vi "Soft_Robot_Model2.vi"() -> ()   [LabVIEW 2015]
uses:
  <vilib>/addons/Control Design/_Model Construction/Model Typedefs.llb/CD State Space Model (MIMO).ctl
  <vilib>/addons/Control Design/_Model Construction/Model Typedefs.llb/CD General Elements.ctl
  <vilib>/Platform/TimedLoop/XDataNode/timing_clust.ctl
  <vilib>/Platform/TimedLoop/XDataNode/nitl_modes.ctl
  <vilib>/Platform/TimedLoop/XDataNode/wakeup.ctl
  <vilib>/addons/Control Design/_Stochastic Systems/Stochastic Systems.llb/Stochastic Systems SubVIs/cd_Stochastic State-Space Model.ctl
  <vilib>/addons/Control Design/_Stochastic Systems/Stochastic Systems.llb/Stochastic Systems SubVIs/cd_Second-Order Statistics Noise Model.ctl
  <vilib>/addons/Control Design/_Model Construction/Model Creation.llb/Model Creation SubVI/cd_Create State Space Model.vi
  <vilib>/Simulation/Estimation/Implementation/NILVSim Discrete Kalman Filter.llb/SIM Disc KF Pred and Corr with Pred Gain with Checking Direct LV.vi
  <vilib>/addons/Control Design/_Implementation/CD State Feedback Controller (Multiple Outputs).vi
  <vilib>/FPGAPlugInAG/myRIO-1900/niLvFpga_Open_myRIO-1900.vi
  <vilib>/rvi/interface/common/dynamic/niFpgaDynamicAddResources.vi
  <vilib>/Utility/error.llb/Error Cluster From Error Code.vi
  <vilib>/rvi/errors/niLvFpgaAdjustHostInterfaceError.vi
  <vilib>/FPGAPlugInAG/Dynamic/niLvFpga_Close_Dynamic.vi
  <vilib>/Platform/TimedLoop/XDataNode/XDataNode.xnode
  <vilib>/Simulation/Implementation/XNodeFramework/SimXNode/SimX.xnode
  <vilib>/rvi/interface/nirviOpenFPGA/nirviOpenFPGA.xnode
  FPGA Bitfiles/ACC20115_FPGATarget_CurrentControlle_Dt5vFgOzYtY.lvbitx
  Current Controller.vi
  <vilib>/rvi/interface/nirviReadWriteControl/nirviReadWriteControl.xnode
  <vilib>/rvi/interface/nirviCloseFPGA/nirviCloseFPGA.xnode
  <vilib>/addons/Control Design/_Model Construction/NI_LinSys_Model Creation.lvlib
  <vilib>/Platform/TimedLoop/XDataNode/XDNodeRunTimeDep.lvlib
  NiFpgaLv.dll
  <vilib>/rvi/interface/Simulation/niFpgaSimulationCallBeginRW.vi
  <vilib>/addons/Control Design/_Implementation/NI_CD_Implementation.lvlib
  <vilib>/addons/Control Design/_Stochastic Systems/NI_CD_Stochastic Systems.lvlib
  <vilib>/addons/Control Design/_Model Construction/NI_LinSys_Model Typedefs.lvlib
panel:
  in  "SP":dbl(slide) scale=0.0..100.0
  in  "Tab Control":enum32{"Outputs", "Inputs"}(tab)
  out "Fusion Data":dbl(graph)
  out "KF Post":dbl[](graph)
  in  "Stop":bool
  out "DAC Inlet Valve 2":i32(graph)
  in  "Current (mA)":i32
  out "Status?":bool
  out "State-Space Model":T1={"properties"={"Model name"="", "Input names"=[], "Output names"=[], "Input Delays"=[], "Output Delays"=[], "Sampling Time"=0.0, "Notes"=""}, "A"=[], "B"=[[3.03e-07], [4.04e-07]], "C"=[], "D"=[], "StateNames"=[], "Transport Delay"=[]} {"Transport Delay" format="%.2f"; "D" format="%#.2g"; "C" format="%#.2g"; "B" format="%#.2g"; "A" format="%#.2g"; "properties"."Sampling Time" format="%#.6p"; "properties"."Output Delays" format="%.4f"; "properties"."Input Delays" format="%.4f"}
  out "KF Gain M(k)":dbl[][](array[numeric])
  in  "A":dbl[][](array[numeric])=[[1.01, -0.1716], [0.001556, 0.9782]] format="%#.5g"
  in  "B":dbl[][](array[numeric]) format="%#.5g"
  in  "C":dbl[][](array[numeric])=[[1.089, -0.03769]] format="%#.5g"
  out "error out":errorcluster
  out "KF Error":errorcluster
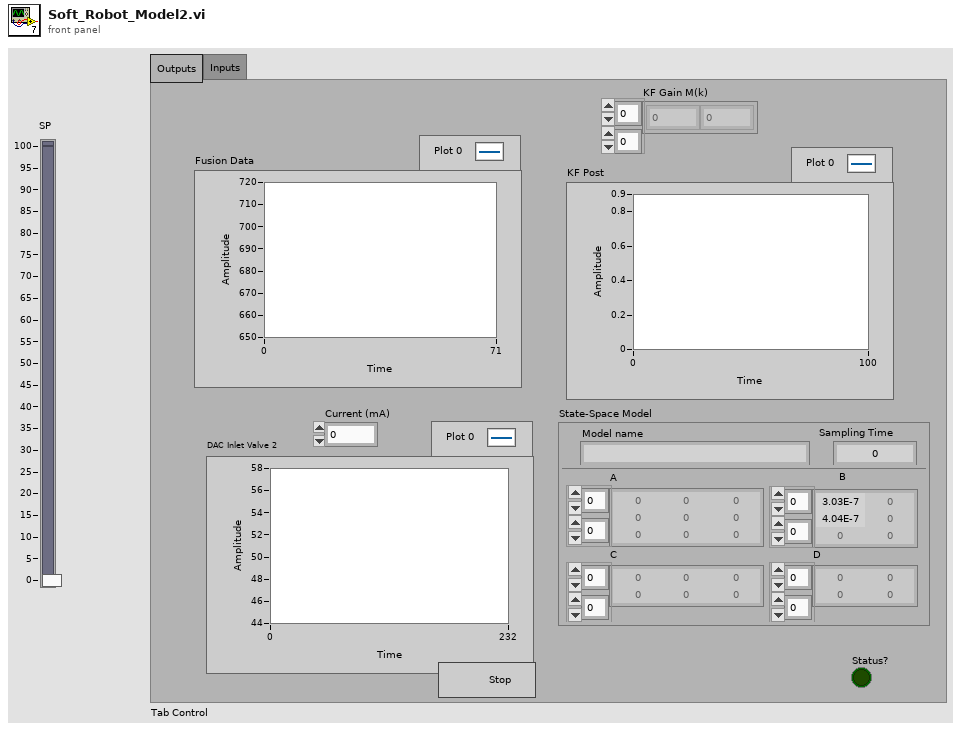
[diagram p1: front panel]
types:
  T1 = typedef "NI_LinSys_Model Typedefs.lvlib/CD State Space Model (MIMO).ctl" = cluster{"properties":T2, "A":dbl[][], "B":dbl[][], "C":dbl[][], "D":dbl[][], "StateNames":string[], "Transport Delay":dbl[][]}
  T2 = typedef "NI_LinSys_Model Typedefs.lvlib/CD General Elements.ctl" = cluster{"Model name":string, "Input names":string[], "Output names":string[], "Input Delays":dbl[], "Output Delays":dbl[], "Sampling Time":dbl, "Notes":string}
  T3 = typedef "XDNodeRunTimeDep.lvlib/timing_clust.ctl" = cluster{"Expected End [f-1]":u64, "Actual End [f-1]":u64, "Finished Late? [f-1]":bool, "Expected End [i-1]":u64, "Actual End [i-1]":u64, "Finished Late? [i-1]":bool, "Expected Start [i]":u64, "Actual Start [i]":u64, "Expected Start [f]":u64, "Actual Start [f]":u64, "Source Name":string, "Structure Name":string, "Period":i64, "Deadline":i64, "Offset":i64, "Start":i64, "Priority":i32, "Timeout":i32, "Mode":T4, "Wakeup Reason":T5, "Error":errorcluster, "Source Type":string, "Secondary Source Type":string, "Global End Time":u64, "Global Start Time":u64, "Frame Duration":u64, "Iteration Duration":u64, "Assigned CPU":i32, "I/O Scan Engine Mode":u32}
  T4 = typedef "XDNodeRunTimeDep.lvlib/nitl_modes.ctl" = enum32{"No Change", "Process missed periods, maintain original phase", "Discard missed periods, maintain original phase", "Process missed periods, ignore original phase", "Discard missed periods, ignore original phase"}
  T5 = typedef "XDNodeRunTimeDep.lvlib/wakeup.ctl" = enum32{"Normal", "Aborted", "Asynchronous wakeup", "Timing source error", "Timed loop error", "Timeout"}
  T6 = typedef "NI_CD_Stochastic Systems.lvlib/cd_Second-Order Statistics Noise Model.ctl" = cluster{"Q":dbl[][], "E{w}":dbl[], "E{v}":dbl[], "R":dbl[][], "N":dbl[][]}
  T7 = typedef "NI_CD_Stochastic Systems.lvlib/cd_Stochastic State-Space Model.ctl" = cluster{"Sampling Time (s)":dbl, "G":dbl[][], "B":dbl[][], "A":dbl[][], "C":dbl[][], "D":dbl[][], "H":dbl[][]}
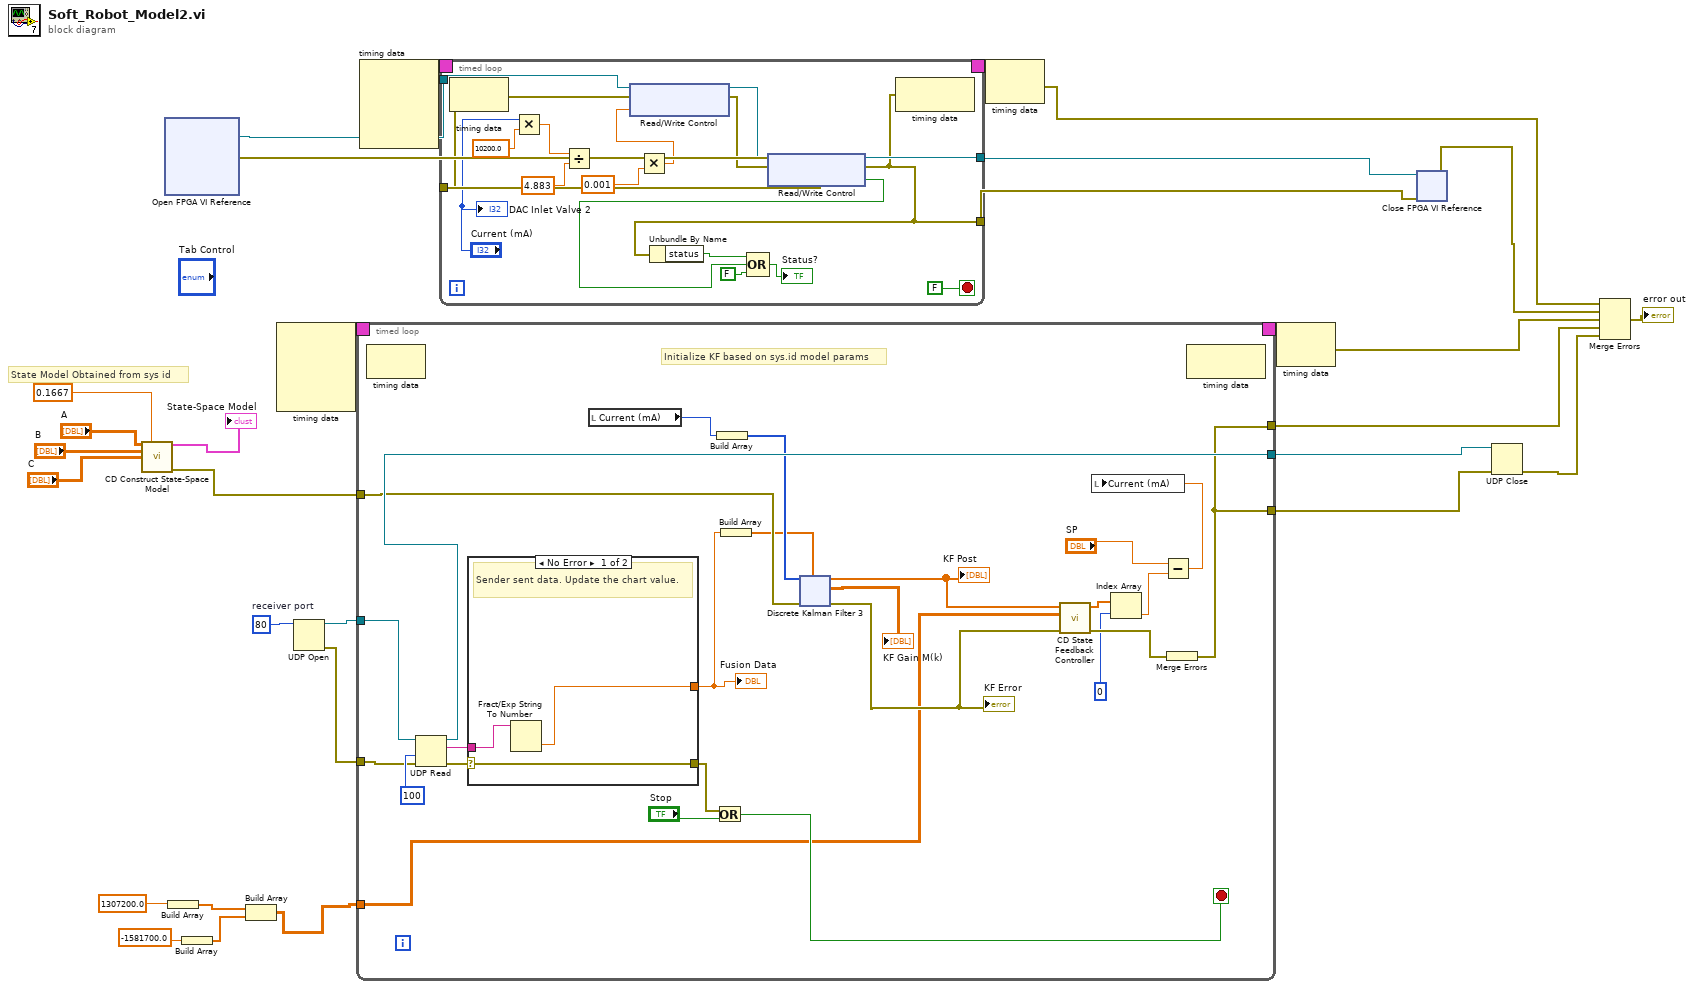
[diagram p0: block diagram]
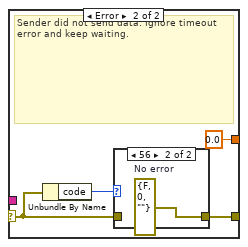
[diagram p2: hidden frame]
diagram:
  w29 = u16 80  # receiver port
  # "State Model Obtained from sys id"
  n1 = call-poly <vilib>:"CD Construct State-Space Model.vi"("A"="A", "Sampling Time (s)"=0.1667, "B"="B", "C"="C") -> ("State-Space Model"=→"State-Space Model":T1, "error out"=w6:errorcluster)  [unwired: 10 in]
  n2 = xnode "Open FPGA VI Reference"() -> ("FPGA VI Reference Out"=w22:refnum<k20>, "error out"=w21:errorcluster)  [unwired: 2 in]
  n3 = Build Array(1307200.0 ("element")) -> (w3:dbl[])
  n4 = Build Array(-1581700.0 ("element")) -> (w2:dbl[])
  n5 = Build Array(w3, w2) -> (w1:dbl[][])
  n6 = node-c288() -> (w24:T3)  [unwired: 4 in]
  n7 = UDP Open(11:w29) -> (port=w28:refnum<k16>, 0:w27:errorcluster)  [unwired: 4 in, 1 out]
  n8 = timed-loop {
    tunnel: [w36] -> w10
    tunnel: w28 -> [w50]
    tunnel: w27 -> [w49]
    tunnel: [w47] -> w26
    timing: w24 -> [_]
    timing-out: [_] -> w23
    tunnel: [w36] -> w18
    tunnel: w6 -> [w44]
    tunnel: w1 -> [w35]
    stop <- w48 stop-if-true
    # "Initialize KF based on sys.id model params"
    n9 = node-c288() -> ()  [unwired: 1 in, 1 out]
    n10 = UDP Read(connection ID=w50, timeout ms (25000)=100, 8:w49) -> (data out=w52:string, error out=w51:errorcluster, 3:w47:refnum<k16>)  [unwired: 3 out]
    n11 = case shown="No Error" w51 {
      selector: w51 -> [w59 w63]
      tunnel: w52 -> [w60 _]
      tunnel: [w59 w62] -> w46
      tunnel: [w58 0.0] -> w40
      frame No Error {
        # "Sender sent data. Update the chart value."
        n12 = Fract/Exp String To Number(string=w60) -> (number=w58:dbl)  [unwired: 3 in, 1 out]
      }
      frame Error {
        # "Sender did not send data. Ignore timeout error and keep waiting."
        n13 = Unbundle By Name(w63) -> ("code"=w64:i32)
        n14 = case shown="56" w64 {
          tunnel: w63 -> [w65 _]
          tunnel: [w65 w66] -> w62
          frame Default {
          }
          frame 56 {
            w66 = errorcluster {"status"=FALSE, "code"=0, "source"=""}  # No error
          }
        }
      }
    }
    "Fusion Data" <- w40
    n15 = local read "Current (mA)"() -> (w55:i32)
    n16 = Or(x=w46, y="Stop") -> (x .or. y?=w48:bool)
    n17 = Build Array ("Build Array 5")(w55) -> (w41:i32[])
    n18 = Build Array ("Build Array 6")(w40) -> (w39:dbl[])
    n19 = xnode ("Discrete Kalman Filter 3")("input u(k)"=w41, "Output y(k)"=w39, "error in (no error)"=w44) -> ("Corrected State Estimate xhat(k|k)"=w31:dbl[], "Kalman Filter Gain M(k)"=→"KF Gain M(k)":dbl[][], "error out"=w42:errorcluster)  [unwired: 5 out]
    "KF Post" <- w31
    "KF Error" <- w42
    n20 = call-poly <vilib>:"CD State Feedback Controller.vi"("error in (no error)"=w42, "Controller Gain"=w35, "States"=w31) -> ("error out"=w43:errorcluster, "Controller Action"=w38:dbl[])  [unwired: 7 in]
    n21 = Index Array(array=w38, index=0) -> (element=w34:dbl)
    n22 = Subtract(x="SP", y=w34) -> (x-y=w33:dbl)
    n23 = local write "Current (mA)"(w33) -> ()
    n24 = Merge Errors(w43) -> (w36:errorcluster)
    n25 = node-c288() -> ()  [unwired: 1 in, 1 out]
  }
  n26 = node-c288() -> (w20:T3)  [unwired: 4 in]
  n27 = timed-loop {
    tunnel: w22 -> [w98]
    tunnel: w21 -> [w83]
    tunnel: [w82] -> w12
    tunnel: [w91] -> w30
    timing: w20 -> [_]
    timing-out: [_] -> w19
    stop <- FALSE stop-if-true
    n28 = node-c288() -> ()  [unwired: 1 in, 1 out]
    n29 = Multiply(x="Current (mA)", y=10200.0) -> (x*y=w86:dbl)
    n30 = Divide(x=w86, y=4.883) -> (x/y=w89:dbl)
    n31 = Multiply(x=w89, y=0.001) -> (x*y=w85:dbl)
    n32 = xnode "Read/Write Control"("FPGA VI Reference In"=w98, "error in"=w83, "DAC Inlet Valve"=w85) -> ("FPGA VI Reference Out"=w97:refnum<k20>, "error out"=w96:errorcluster)
    n33 = xnode "Read/Write Control"("FPGA VI Reference In"=w97, "error in"=w96) -> ("FPGA VI Reference Out"=w91:refnum<k20>, "error out"=w82:errorcluster, "Inlet Overflow?"=w92:bool)
    n34 = Unbundle By Name(w82) -> ("status"=w94:bool)
    n35 = Compound Arithmetic op=OR(w94, w92, FALSE ("value")) -> (→"Status?":bool)
    n36 = node-c288(w82) -> ()  [unwired: 1 out]
    "DAC Inlet Valve 2" <- "Current (mA)"
  }
  n37 = node-c288(w19) -> (w7:errorcluster)
  n38 = node-c288(w23) -> (w9:errorcluster)
  n39 = xnode "Close FPGA VI Reference"("FPGA VI Reference In"=w30, "error in"=w12) -> ("error out"=w8:errorcluster)
  n40 = UDP Close(connection ID=w26, 8:w18) -> (error out=w11:errorcluster)  [unwired: 1 out]
  n41 = Merge Errors(w7, w8, w9, w10, w11) -> (→"error out":errorcluster)
